vi "Post-Process.vi"(11 "Chmmr in":refnum<class "Chmmr.lvclass">) -> (2 "New Elements":refnum<class "Element.lvclass">[](array[class]), 3 "Chmmr out":refnum<class "Chmmr.lvclass">)   [LabVIEW 2021, in "Chmmr.lvclass"]
uses:
  Chmmr.lvclass
  Element/Element.lvclass
  Ship/Ship.lvclass
  Chmmr.lvclass/Chmmr.ctl
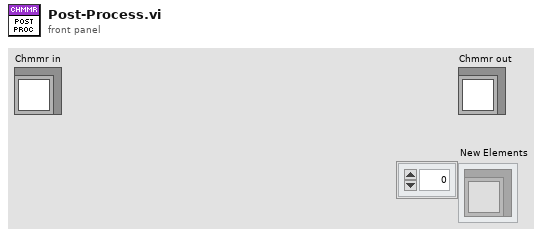
[diagram p1: front panel]
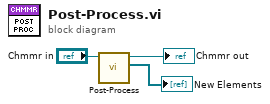
[diagram p0: block diagram]
diagram:
  n1 = call-parent "Post-Process.vi"("Ship in"="Chmmr in") -> ("New Elements"=→"New Elements":refnum<class "Element.lvclass">[], "Ship out"=→"Chmmr out":refnum<class "Chmmr.lvclass">)  [unwired: 9 in]
